vi "GetPointType2D_3D-SGL.vi"(11 "Point":T1) -> (3 "Point":T2)   [LabVIEW 2020, in "OpenLvVision_OpenCv.lvlib"]
uses:
  TypeDef/Point/2D_PointSGL.ctl
  OpenLvVision_OpenCv.lvlib
  TypeDef/Point/3D_PointSGL.ctl
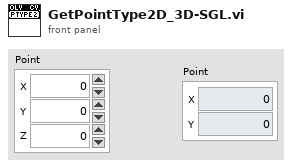
[diagram p1: front panel]
types:
  T1 = typedef "OpenLvVision_OpenCv.lvlib/3D_PointSGL.ctl" = cluster{"X":sgl, "Y":sgl, "Z":sgl}
  T2 = typedef "OpenLvVision_OpenCv.lvlib/2D_PointSGL.ctl" = cluster{"X":sgl, "Y":sgl}
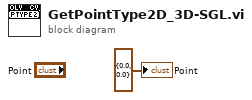
[diagram p0: block diagram]
diagram:
  "Point" <- T2 {"X"=0.0, "Y"=0.0} ("Point")
